vi "Event Handler.vi"(0 "uService Template in":refnum<class "Test_uService.lvclass">, 5 "Event type":T1=enum."Message", 7 "Item Name":string, 9 "Data":variant, 11 "error in (no error)":errorcluster) -> (4 "uService Template out":refnum<class "Test_uService.lvclass">, 15 "error out":errorcluster)   [LabVIEW 2020, in "Test_uService.lvlib" / "Test_uService.lvclass"]
doc: "This VI is the event handler of the uService: every time an event is triggered to the uService, this VI is called.\nNote: here you can access the Actor/Class data, but it will be the one coming out from Init. You cannot modify the values.\nThree different events are supported:\nI) Button Pressed: get called on a GUI button pressed. Item Name is the name (label) of the button, Data is empty.\nII) Shared Variable Updated: get called when a SV you subscribed to is updated. Item Name is the name of the SV, and Data is the value (note: you need to convert it to the proper type).\nIII) Message: get called every time a user event is generated using Send Message to Event Handler. The values of Item Name and Data are the one given to the Send Message to Event Handler.\nIV) Ready to launch?: this frame get called every time a new Run is initiated. Each uService is responsible of performing a self check before giving back the green light for the Run to start."
uses:
  Test_uService.lvclass
  Test_uService.lvclass/Test_uService.ctl
  TALOS/TALOS_PPL.lvlibp
  Test_uService Consumer Case Selector.ctl
  TALOS/TALOS_PPL.lvlibp/Father of all uServices/Father of all uServices/Father of all uServices.lvclass
  C:/LabVIEW Code/aegis-labview-code/TALOS/TALOS_PPL.lvlibp/Father of all uServices/Father of all uServices/Father of all uServices.lvclass
  TALOS/TALOS_PPL.lvlibp/Father of all uServices/Father of all uServices/Event Handler Items.ctl
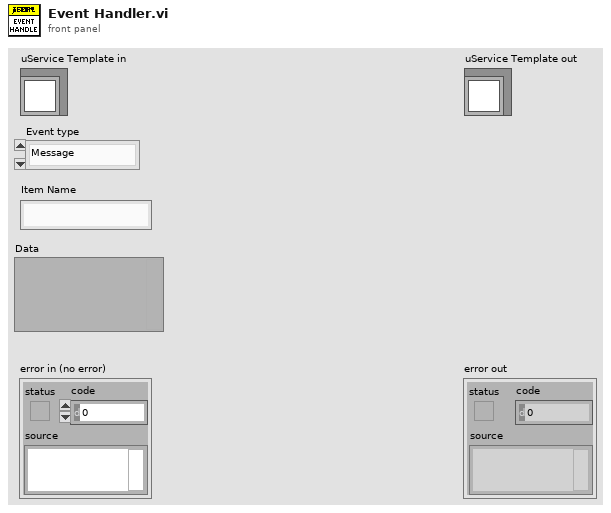
[diagram p1: front panel]
types:
  T1 = typedef "TALOS_PPL.lvlibp/Father of all uServices.lvlib/Father of all uServices.lvclass/Event Handler Items.ctl" = enum16{"Button Pressed", "Message", "Ready to launch?", "Safe Mode", "Start RUN", "Stop RUN"}
  T2 = typedef "Test_uService.lvlib/Test_uService.lvclass/Test_uService Consumer Case Selector.ctl" = enum16{"Start echo", "Echo arrived"}
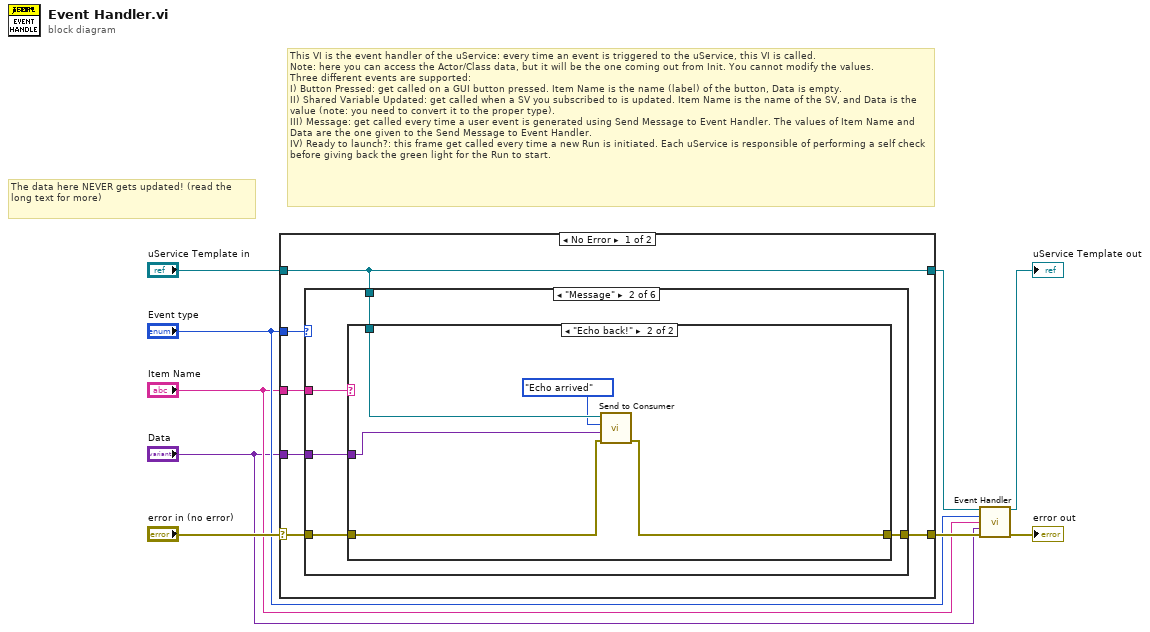
[diagram p0: block diagram]
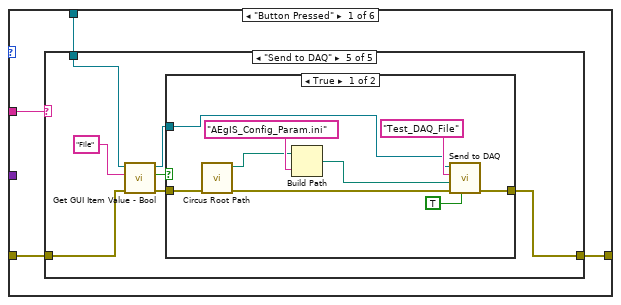
[diagram p2: hidden frame]
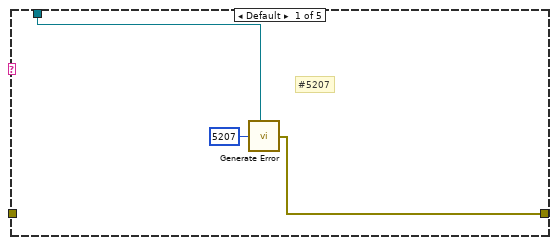
[diagram p3: hidden frame]
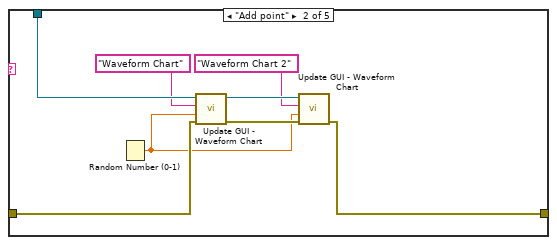
[diagram p4: hidden frame]
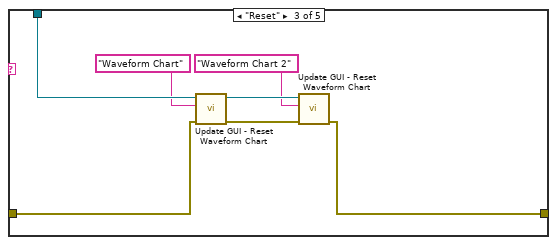
[diagram p5: hidden frame]
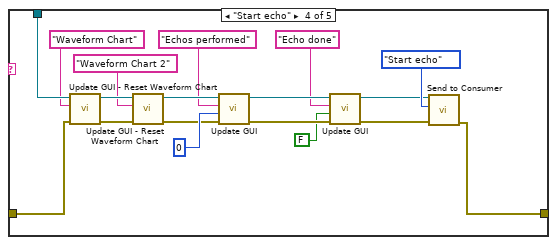
[diagram p6: hidden frame]
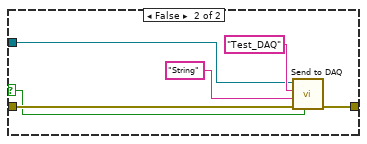
[diagram p7: hidden frame]
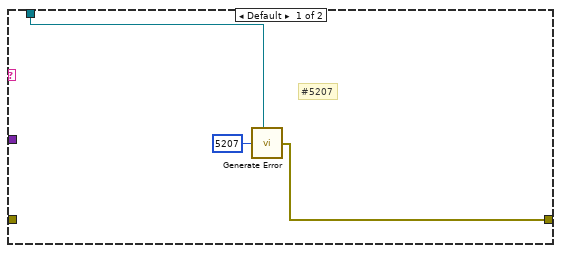
[diagram p8: hidden frame]
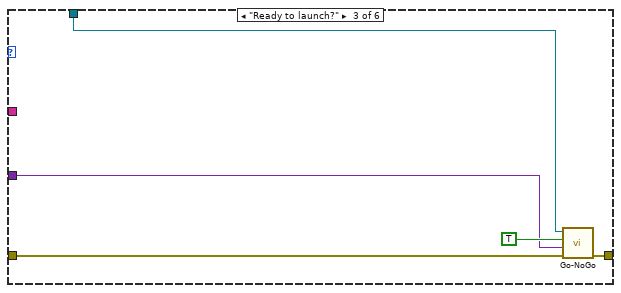
[diagram p9: hidden frame]
diagram:
  # "The data here NEVER gets updated! (read the long text for more)"
  # "This VI is the event handler of the uService: every time an event is triggered to the uService, this VI is called.\nNote: here you can access the Actor/Class data, but it will be the one coming out from Init. You cannot modify the values.\nThree different events are supported:\nI) Button Pressed: get called on a GUI button pressed. Item Name is the name (label) of the button, Data is empty.\nII) Shared Variable Updated: get called when a SV you subscribed to is updated. Item Name is the name of the SV, and Data is the value (note: you need to convert it to the proper type).\nIII) Message: get called every time a user event is generated using Send Message to Event Handler. The values of Item Name and Data are the one given to the Send Message to Event Handler.\nIV) Ready to launch?: this frame get called every time a new Run is initiated. Each uService is responsible of performing a self check before giving back the green light for the Run to start."
  n1 = case shown="No Error" "error in (no error)" {
    selector: "error in (no error)" -> [w13 w100]
    tunnel: [w14 w100] -> w7
    tunnel: [w12 w99] -> w4
    tunnel: "uService Template in" -> [w12 w99]
    tunnel: "Event type" -> [w15 _]
    tunnel: "Item Name" -> [w11 _]
    tunnel: "Data" -> [w10 _]
    frame No Error {
      n2 = case shown="\"Message\"" w15 {
        tunnel: [w19 w78 w94 w96 w97 w98] -> w14
        tunnel: w13 -> [w16 w82 w95 w96 w97 w98]
        tunnel: w11 -> [w17 w81 _ _ _ _]
        tunnel: w12 -> [w18 w79 w93 _ _ _]
        tunnel: w10 -> [_ w80 w91 _ _ _]
        frame "Button Pressed" {
          n3 = case shown="\"Send to DAQ\"" w17 {
            tunnel: w16 -> [_ w27 w34 w53 w60]
            tunnel: [w20 w28 w35 w45 w62] -> w19
            tunnel: w18 -> [w21 w30 w37 w55 w58]
            frame Default {
              # "#5207"
              n4 = call "Generate Error.vi"("Class"=w21, "Error Code"=5207) -> ("error out"=w20:errorcluster)  [unwired: 5 in]
            }
            frame "Add point" {
              n5 = Random Number (0-1)() -> (number: 0 to 1=w23:dbl)
              n6 = call "Update GUI - Waveform Chart.vi"("error in (no error)"=w27, "Point value"=w23, "GUI Item Name"="Waveform Chart", "uService Template in"=w30) -> ("error out"=w26:errorcluster, "uService Template out"=w29:refnum<class "Test_uService.lvclass">)  [unwired: 6 in]
              n7 = call "Update GUI - Waveform Chart.vi"("error in (no error)"=w26, "Point value"=w23, "GUI Item Name"="Waveform Chart 2", "uService Template in"=w29) -> ("error out"=w28:errorcluster)  [unwired: 6 in, 1 out]
            }
            frame "Reset" {
              n8 = call "Update GUI - Reset Waveform Chart.vi"("error in (no error)"=w34, "GUI Item Name"="Waveform Chart", "uService Template in"=w37) -> ("error out"=w33:errorcluster, "uService Template out"=w36:refnum<class "Test_uService.lvclass">)  [unwired: 7 in]
              n9 = call "Update GUI - Reset Waveform Chart.vi"("error in (no error)"=w33, "GUI Item Name"="Waveform Chart 2", "uService Template in"=w36) -> ("error out"=w35:errorcluster)  [unwired: 7 in, 1 out]
            }
            frame "Start echo" {
              n10 = call "Update GUI - Reset Waveform Chart.vi"("error in (no error)"=w53, "GUI Item Name"="Waveform Chart", "uService Template in"=w55) -> ("error out"=w52:errorcluster, "uService Template out"=w54:refnum<class "Test_uService.lvclass">)  [unwired: 7 in]
              n11 = call "Update GUI - Reset Waveform Chart.vi"("error in (no error)"=w52, "GUI Item Name"="Waveform Chart 2", "uService Template in"=w54) -> ("error out"=w46:errorcluster, "uService Template out"=w49:refnum<class "Test_uService.lvclass">)  [unwired: 7 in]
              n12 = call "Update GUI.vi"("error in (no error)"=w46, "Data"=u16 0, "GUI Item Name"="Echos performed", "uService Template in"=w49) -> ("error out"=w40:errorcluster, "uService Template out"=w43:refnum<class "Test_uService.lvclass">)  [unwired: 6 in]
              n13 = call "Update GUI.vi"("error in (no error)"=w40, "Data"=FALSE, "GUI Item Name"="Echo done", "uService Template in"=w43) -> ("error out"=w39:errorcluster, "uService Template out"=w42:refnum<class "Test_uService.lvclass">)  [unwired: 6 in]
              n14 = call "Send to Consumer.vi"("error in (no error)"=w39, "Case ID"=Test_uService_Consumer_Case_Selector."Start echo" ("Consumer Case Selector"), "uService Template in"=w42) -> ("error out"=w45:errorcluster)  [unwired: 7 in, 1 out]
            }
            frame "Send to DAQ" {
              n15 = call "Get GUI Item Value - Bool.vi"("error in (no error)"=w60, "FP Item Name"="File", "uService Template in"=w58) -> ("error out"=w61:errorcluster, "Value"=w57:bool, "uService Template out"=w56:refnum<class "Test_uService.lvclass">)  [unwired: 6 in]
              n16 = case shown="True" w57 {
                selector: w57 -> [_ w75]
                tunnel: [w71 w77] -> w62
                tunnel: w61 -> [w64 w76]
                tunnel: w56 -> [w66 w72]
                frame True {
                  n17 = call "Circus Root Path.vi"("error in (no error)"=w64) -> ("error out"=w65:errorcluster, "Circus Root Path"=w63:path)  [unwired: 9 in]
                  n18 = Build Path(base path=w63, name or relative path="AEgIS_Config_Param.ini") -> (appended path=w67:path)
                  n19 = call "Send to DAQ.vi"("File?"=TRUE, "error in (no error)"=w65, "Data"=w67, "Data Name"="Test_DAQ_File", "Father of all uServices in"=w66) -> ("error out"=w71:errorcluster)  [unwired: 5 in, 1 out]
                }
                frame False {
                  n20 = call "Send to DAQ.vi"("File?"=w75, "error in (no error)"=w76, "Data"="String", "Data Name"="Test_DAQ", "Father of all uServices in"=w72) -> ("error out"=w77:errorcluster)  [unwired: 5 in, 1 out]
                }
              }
            }
          }
        }
        frame "Message" {
          n21 = case shown="\"Echo back!\"" w81 {
            tunnel: w82 -> [_ w88]
            tunnel: w80 -> [_ w86]
            tunnel: w79 -> [w84 w90]
            tunnel: [w83 w87] -> w78
            frame Default {
              # "#5207"
              n22 = call "Generate Error.vi"("Class"=w84, "Error Code"=5207) -> ("error out"=w83:errorcluster)  [unwired: 5 in]
            }
            frame "Echo back!" {
              n23 = call "Send to Consumer.vi"("error in (no error)"=w88, "Data"=w86, "Case ID"=Test_uService_Consumer_Case_Selector."Echo arrived" ("Consumer Case Selector"), "uService Template in"=w90) -> ("error out"=w87:errorcluster)  [unwired: 6 in, 1 out]
            }
          }
        }
        frame "Ready to launch?" {
          n24 = call-dynamic "Go-NoGo.vi"("error in (no error)"=w95, "Go-NoGo Data"=w91, "Go?"=TRUE, "Father of all uServices in"=w93) -> ("error out"=w94:errorcluster)  [unwired: 6 in, 1 out]
        }
        frame "Safe Mode" {
        }
        frame "Start RUN" {
        }
        frame "Stop RUN" {
        }
      }
    }
    frame Error {
    }
  }
  n25 = call-parent "Event Handler.vi"("uService Template in"=w4, "Event type"="Event type", "Item Name"="Item Name", "Data"="Data", "error in (no error)"=w7) -> ("uService Template out"=→"uService Template out":refnum<class "Test_uService.lvclass">, "error out"=→"error out":errorcluster)  [unwired: 9 in]
